vi "BoolConfirmCheck.vi"(2 "False Time":dbl, 3 "Secondary True Time":dbl, 4 "Inital True Time":dbl, 5 "Signal":bool) -> (0 "First Time Met":bool, 1 "Out Signal":bool)   [LabVIEW 2016]
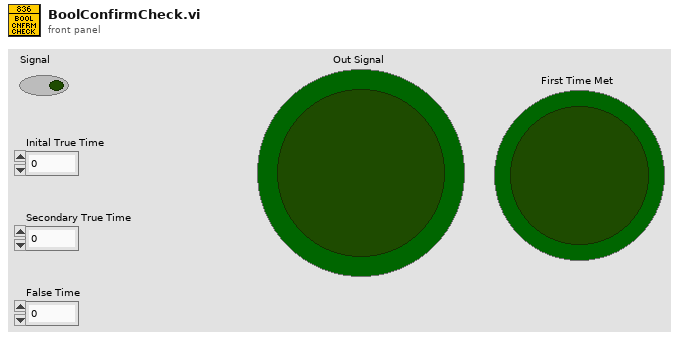
[diagram p1: front panel]
types:
  T1 = enum16{"idle", "initial", "inbetween", "secondary"}
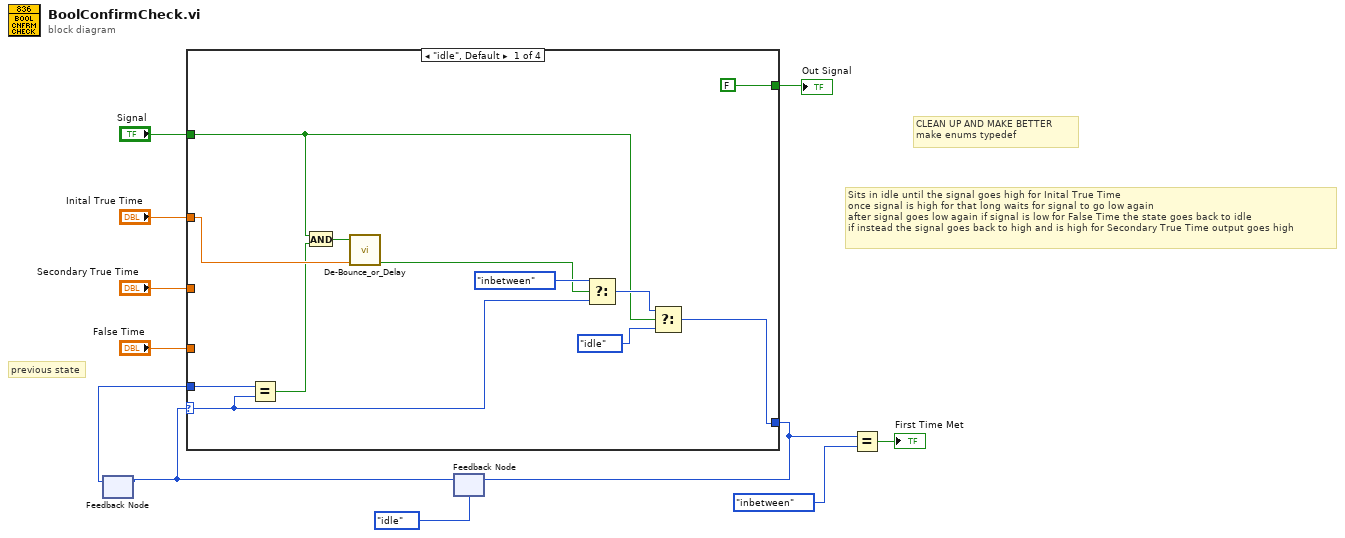
[diagram p0: block diagram]
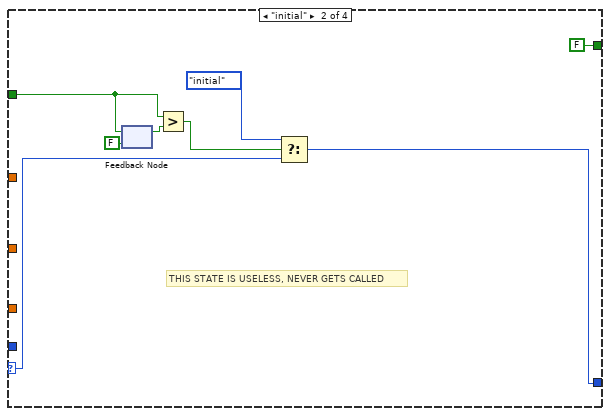
[diagram p2: hidden frame]
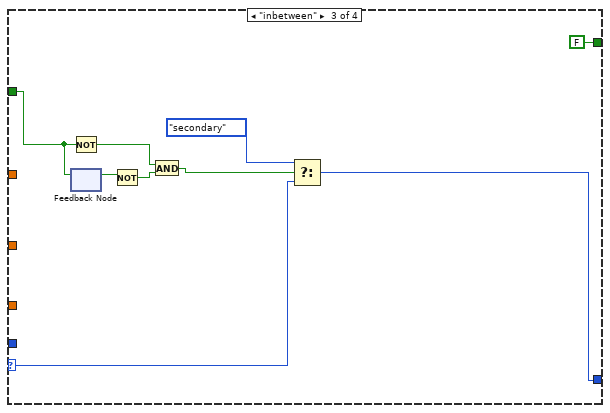
[diagram p3: hidden frame]
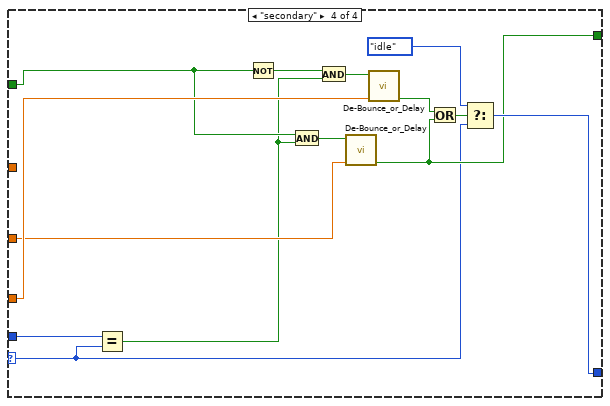
[diagram p4: hidden frame]
diagram:
  # "Sits in idle until the signal goes high for Inital True Time\nonce signal is high for that long waits for signal to go low again\nafter signal goes low again if signal is low for False Time the state goes back to idle\nif instead the signal goes back to high and is high for Secondary True Time output goes high"
  # "CLEAN UP AND MAKE BETTER\nmake enums typedef"
  # "previous state"
  n1 = feedback #1() -> (w4:T1)  [unwired: 1 in]
  n2 = feedback #2(T1."idle") -> (w5:T1)
  n3 = feedback-in #1(w5) -> ()
  n4 = case shown="\"idle\", Default" w5 {
    selector: w5 -> [w12 w27 w37 w42]
    tunnel: [w18 w25 w40 w52] -> w3
    tunnel: "Signal" -> [w15 w31 w36 w44]
    tunnel: "Inital True Time" -> [w20 _ _ _]
    tunnel: "Secondary True Time" -> [_ _ _ w49]
    tunnel: "False Time" -> [_ _ _ w54]
    tunnel: [FALSE ("Out Signal") FALSE ("Out Signal") FALSE ("Out Signal") w48] -> w6
    tunnel: w4 -> [w14 _ _ w43]
    frame "idle", Default {
      n5 = Equal?(x=w14, y=w12) -> (x = y?=w13:bool)
      n6 = And(x=w15, y=w13) -> (x .and. y?=w16:bool)
      n7 = call <userlib>:"De-Bounce_or_Delay.vi"("Eval Period (sec)"=w20, "Signal Input"=w16) -> ("Stable"=w19:bool)  [unwired: 9 in]
      n8 = Select(t=T1."inbetween", s=w19, f=w12) -> (s? t:f=w21:T1)
      n9 = Select(t=w21, s=w15, f=T1."idle") -> (s? t:f=w18:T1)
    }
    frame "initial" {
      # "THIS STATE IS USELESS, NEVER GETS CALLED"
      n10 = feedback-in #3(w31) -> ()
      n11 = feedback #3(FALSE ("Signal")) -> (w30:bool)
      n12 = Greater?(x=w31, y=w30) -> (0:w28:bool)
      n13 = Select(t=T1."initial", s=w28, f=w27) -> (s? t:f=w25:T1)
    }
    frame "inbetween" {
      n14 = Not(x=w36) -> (.not. x?=w33:bool)
      n15 = feedback-in #4(w36) -> ()
      n16 = feedback #4() -> (w35:bool)  [unwired: 1 in]
      n17 = Not(x=w35) -> (.not. x?=w34:bool)
      n18 = And(x=w33, y=w34) -> (x .and. y?=w32:bool)
      n19 = Select(t=T1."secondary" ("f"), s=w32, f=w37) -> (s? t:f=w40:T1)
    }
    frame "secondary" {
      n20 = Equal?(x=w43, y=w42) -> (x = y?=w41:bool)
      n21 = Not(x=w44) -> (.not. x?=w46:bool)
      n22 = And(x=w44, y=w41) -> (x .and. y?=w45:bool)
      n23 = And(x=w46, y=w41) -> (x .and. y?=w47:bool)
      n24 = call <userlib>:"De-Bounce_or_Delay.vi"("Eval Period (sec)"=w49, "Signal Input"=w45) -> ("Stable"=w48:bool)  [unwired: 9 in]
      n25 = call <userlib>:"De-Bounce_or_Delay.vi"("Eval Period (sec)"=w54, "Signal Input"=w47) -> ("Stable"=w51:bool)  [unwired: 9 in]
      n26 = Or(x=w51, y=w48) -> (x .or. y?=w50:bool)
      n27 = Select(t=T1."idle", s=w50, f=w42) -> (s? t:f=w52:T1)
    }
  }
  "Out Signal" <- w6
  n28 = feedback-in #2(w3) -> ()
  n29 = Equal?(x=w3, y=T1."inbetween") -> (x = y?=→"First Time Met":bool)
